vi "UDP Receiver.vi"(0 "IP Adress":string="10.0.136.51", 1 "Port":u16=1234) -> (7 "Accelerometer Data":cluster{"X":dbl, "Y":dbl, "Z":dbl}, 10 "Output Errors":errorcluster)   [LabVIEW 2019]
panel:
  out "appended array":dbl[][](array[numeric])
  out "Array":string="1395245468255282000; -0.8595; -0.0790; 9.6929; -0.6874; -5.4853; -0.3169; 22.00; -17.80; -34.10; 1017.7800"
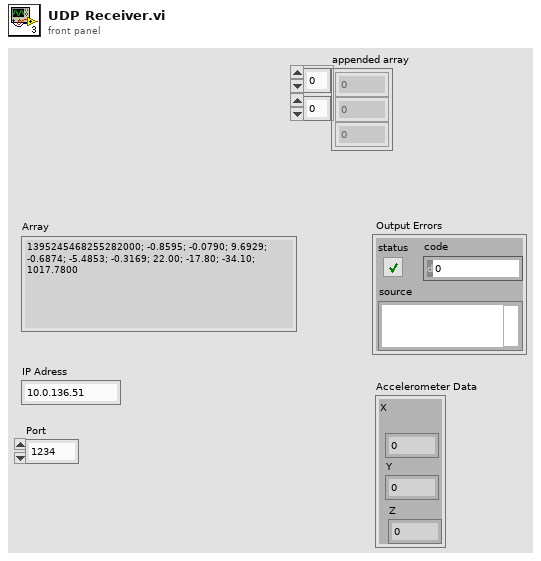
[diagram p1: front panel]
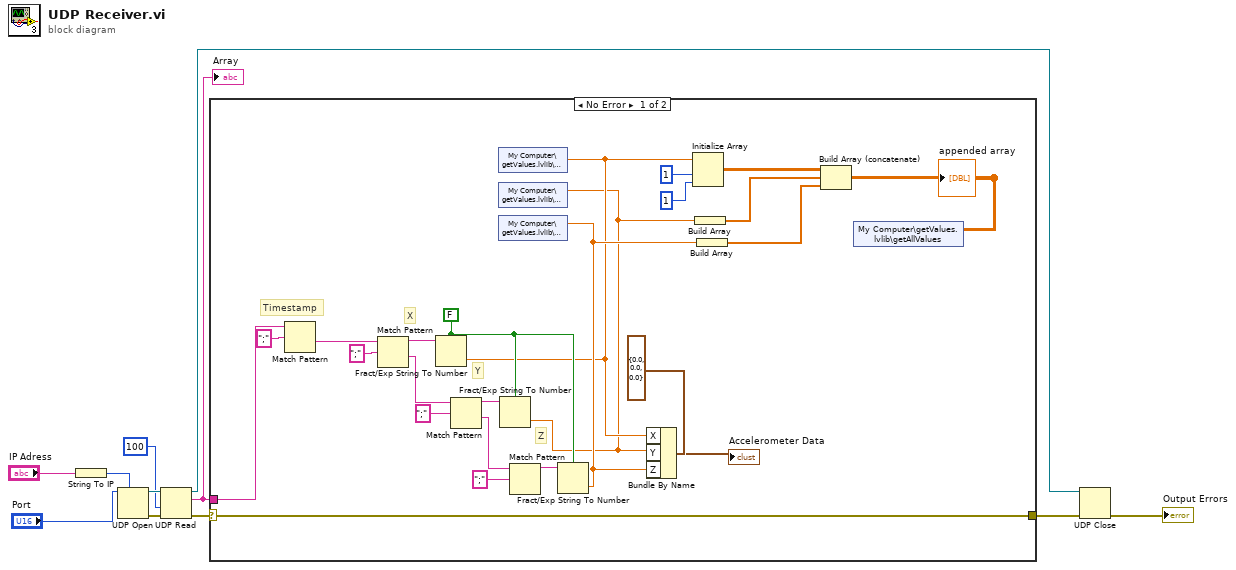
[diagram p0: block diagram]
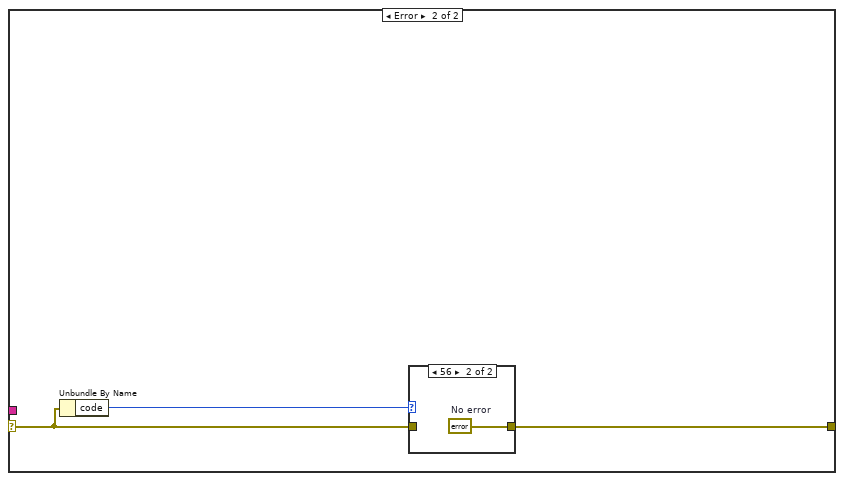
[diagram p2: hidden frame]
diagram:
  n1 = String To IP(1:"IP Adress") -> (0:w8:u32)
  n2 = UDP Open(7:w8, 11:"Port") -> (port=w9:refnum<k16>, 0:w10:errorcluster)  [unwired: 3 in, 1 out]
  n3 = UDP Read(connection ID=w9, timeout ms (25000)=100, 8:w10) -> (data out=w2:string, error out=w3:errorcluster, 3:w1:refnum<k16>)  [unwired: 3 out]
  "Array" <- w2
  n4 = case shown="No Error" w3 {
    selector: w3 -> [w35 w37]
    tunnel: w2 -> [w34 _]
    tunnel: [w35 w36] -> w11
    frame No Error {
      w23 = FALSE ("utiliser le séparateur décimal du système (V)")
      # "Timestamp"
      # "Z"
      # "Y"
      # "X"
      n5 = Match Pattern(string=w34, regular expression=";" ("expression régulière")) -> (after substring=w31:string)  [unwired: 1 in, 3 out]
      n6 = Match Pattern(string=w31, regular expression=";" ("expression régulière")) -> (before substring=w30:string, after substring=w28:string)  [unwired: 1 in, 2 out]
      n7 = Fract/Exp String To Number(use system decimal point (T)=w23, string=w30) -> (number=w13:dbl)  [unwired: 2 in, 1 out]
      n8 = Match Pattern(string=w28, regular expression=";" ("expression régulière")) -> (before substring=w27:string, after substring=w25:string)  [unwired: 1 in, 2 out]
      n9 = shared-variable "My Computer\\getValues.lvlib\\getX"(w13) -> ()  [unwired: 1 in, 1 out]
      n10 = Fract/Exp String To Number(use system decimal point (T)=w23, string=w27) -> (number=w12:dbl)  [unwired: 2 in, 1 out]
      n11 = shared-variable "My Computer\\getValues.lvlib\\getY"(w12) -> ()  [unwired: 1 in, 1 out]
      n12 = Match Pattern(string=w25, regular expression=";" ("expression régulière")) -> (before substring=w24:string)  [unwired: 1 in, 3 out]
      n13 = Fract/Exp String To Number(use system decimal point (T)=w23, string=w24) -> (number=w18:dbl)  [unwired: 2 in, 1 out]
      n14 = shared-variable "My Computer\\getValues.lvlib\\getZ"(w18) -> ()  [unwired: 1 in, 1 out]
      n15 = Bundle By Name(cluster=cluster{"X":dbl, "Y":dbl, "Z":dbl} {"X"=0.0, "Y"=0.0, "Z"=0.0} ("input cluster"), "X"=w13, "Y"=w12, "Z"=w18) -> (→"Accelerometer Data":cluster{"X":dbl, "Y":dbl, "Z":dbl})
      n16 = Initialize Array(w13, 1, 1) -> (w17:dbl[][])
      n17 = Build Array(w12) -> (w16:dbl[])
      n18 = Build Array(w18) -> (w15:dbl[])
      n19 = Build Array (concatenate)(w17, w16, w15) -> (w14:dbl[][])
      "appended array" <- w14
      n20 = shared-variable "My Computer\\getValues.lvlib\\getAllValues"(w14) -> ()  [unwired: 1 in, 1 out]
    }
    frame Error {
      # "L'émetteur n'a pas envoyé de données. Ignorer l'erreur de timeout et continuer à attendre."
      n21 = Unbundle By Name(w37) -> ("code"=w38:i32)
      n22 = case shown="56" w38 {
        tunnel: w37 -> [w39 _]
        tunnel: [w39 w40] -> w36
        frame Default {
        }
        frame 56 {
          w40 = errorcluster {"status"=FALSE, "code"=0, "source"=""}  # No error
        }
      }
    }
  }
  n23 = UDP Close(connection ID=w1, 8:w11) -> (error out=→"Output Errors":errorcluster)  [unwired: 1 out]
